vi "Configure Trigger Link.vi"(0 "VISA resource name":refnum<visa-resource-name>, 1 "Trigger Layer Input Port (3)":u32=3, 2 "Trigger Layer Output Port (4)":u32=4, 5 "Arm Layer Input Port (1)":u32=1, 7 "Arm Layer Output Port (2)":u32=2, 9 "Arm Layer Output Events (1)":u32=1, 11 "error in (no error)":errorcluster, 12 "Trigger Layer Input Events (1)":u32=1, 13 "Trigger Layer Output Events (1)":u32=1) -> (4 "VISA resource name out":refnum<visa-resource-name>, 15 "error out":errorcluster)   [LabVIEW 2012, in "Keithley 24XX.lvlib"]
doc: "Configure the trigger link ports as well as the events that require or create a trigger event."
uses:
  <instrlib>/Keithley 24XX/Keithley 24XX.lvlib
panel:
  # "Arm Layer Controls"
  # "Trigger Layer Controls"
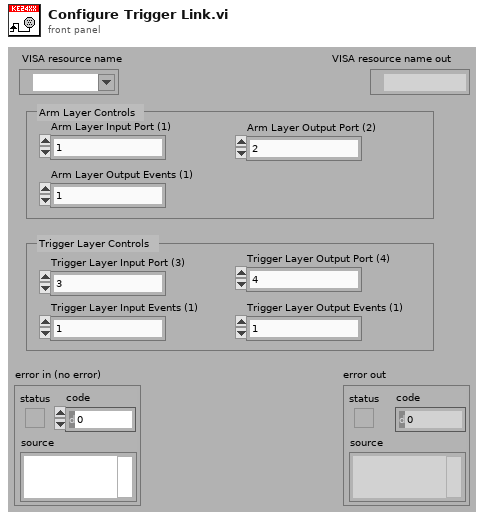
[diagram p1: front panel]
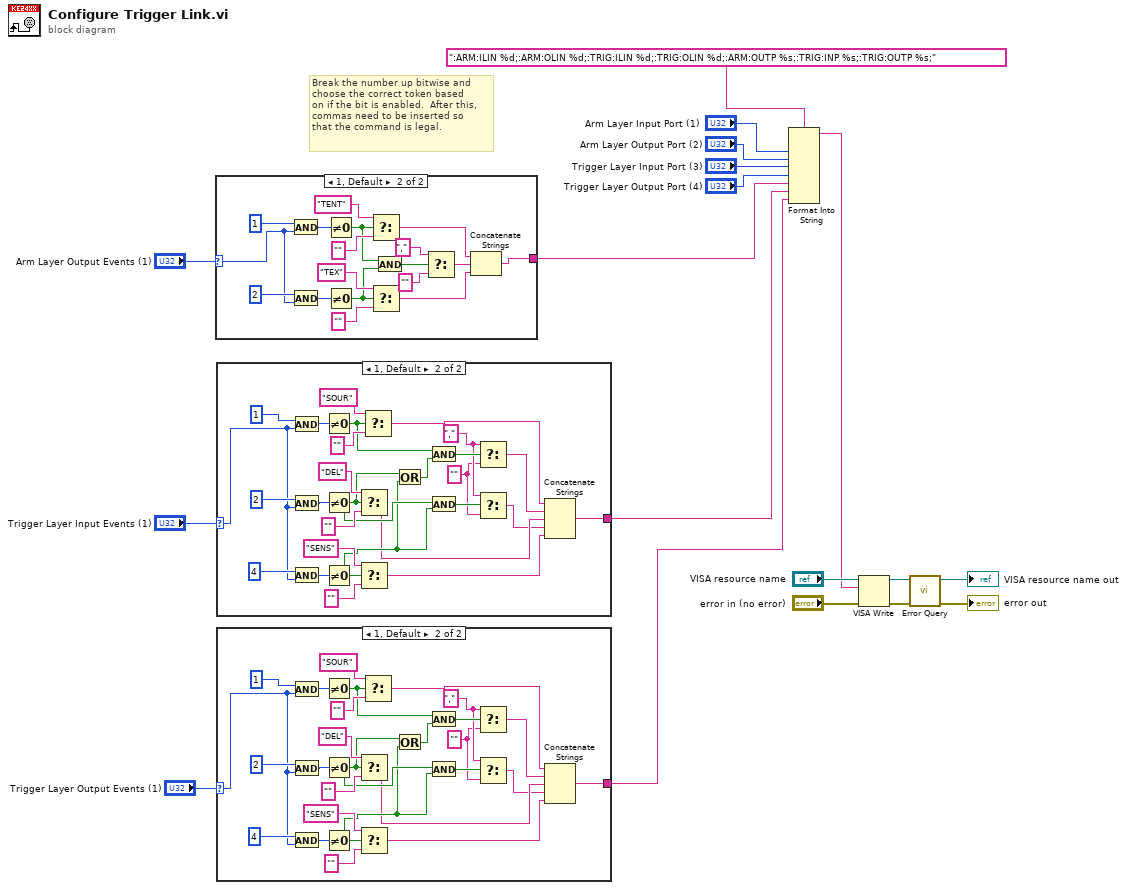
[diagram p0: block diagram]
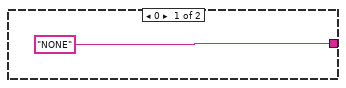
[diagram p2: hidden frame]
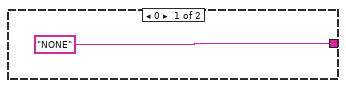
[diagram p3: hidden frame]
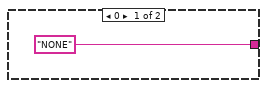
[diagram p4: hidden frame]
diagram:
  # "Break the number up bitwise and\nchoose the correct token based\non if the bit is enabled.  After this, \ncommas need to be inserted so \nthat the command is legal."
  n1 = case shown="1, Default" "Arm Layer Output Events (1)" {
    selector: "Arm Layer Output Events (1)" -> [_ w35]
    tunnel: ["NONE" w20] -> w4
    frame 0 {
    }
    frame 1, Default {
      n2 = And(x=1, y=w35) -> (x .and. y?=w34:u32)
      n3 = And(x=2, y=w35) -> (x .and. y?=w33:u32)
      n4 = Not Equal To 0?(x=w34) -> (x != 0?=w28:bool)
      n5 = Not Equal To 0?(x=w33) -> (x != 0?=w27:bool)
      n6 = Select(t="TENT", s=w28, f="") -> (s? t:f=w21:string)
      n7 = Select(t="TEX", s=w27, f="") -> (s? t:f=w22:string)
      n8 = And(x=w28, y=w27) -> (x .and. y?=w26:bool)
      n9 = Select(t=",", s=w26, f="") -> (s? t:f=w23:string)
      n10 = Concatenate Strings(w21, w23, w22) -> (w20:string)
    }
  }
  n11 = case shown="1, Default" "Trigger Layer Input Events (1)" {
    selector: "Trigger Layer Input Events (1)" -> [_ w62]
    tunnel: ["NONE" w39] -> w3
    frame 0 {
    }
    frame 1, Default {
      w46 = ","
      w45 = ""
      n12 = And(x=1, y=w62) -> (x .and. y?=w60:u32)
      n13 = And(x=2, y=w62) -> (x .and. y?=w61:u32)
      n14 = And(x=4, y=w62) -> (x .and. y?=w59:u32)
      n15 = Not Equal To 0?(x=w60) -> (x != 0?=w52:bool)
      n16 = Not Equal To 0?(x=w61) -> (x != 0?=w50:bool)
      n17 = Not Equal To 0?(x=w59) -> (x != 0?=w49:bool)
      n18 = Select(t="DEL", s=w50, f="") -> (s? t:f=w42:string)
      n19 = Select(t="SENS", s=w49, f="") -> (s? t:f=w40:string)
      n20 = Select(t="SOUR", s=w52, f="") -> (s? t:f=w44:string)
      n21 = Or(x=w50, y=w49) -> (x .or. y?=w51:bool)
      n22 = And(x=w52, y=w51) -> (x .and. y?=w48:bool)
      n23 = And(x=w50, y=w49) -> (x .and. y?=w47:bool)
      n24 = Select(t=w46, s=w48, f=w45) -> (s? t:f=w43:string)
      n25 = Select(t=w46, s=w47, f=w45) -> (s? t:f=w41:string)
      n26 = Concatenate Strings(w44, w43, w42, w41, w40) -> (w39:string)
    }
  }
  n27 = case shown="1, Default" "Trigger Layer Output Events (1)" {
    selector: "Trigger Layer Output Events (1)" -> [_ w90]
    tunnel: ["NONE" w67] -> w1
    frame 0 {
    }
    frame 1, Default {
      w74 = ","
      w73 = ""
      n28 = And(x=1, y=w90) -> (x .and. y?=w88:u32)
      n29 = And(x=2, y=w90) -> (x .and. y?=w89:u32)
      n30 = And(x=4, y=w90) -> (x .and. y?=w87:u32)
      n31 = Not Equal To 0?(x=w88) -> (x != 0?=w80:bool)
      n32 = Not Equal To 0?(x=w89) -> (x != 0?=w78:bool)
      n33 = Not Equal To 0?(x=w87) -> (x != 0?=w77:bool)
      n34 = Select(t="DEL", s=w78, f="") -> (s? t:f=w70:string)
      n35 = Select(t="SENS", s=w77, f="") -> (s? t:f=w68:string)
      n36 = Select(t="SOUR", s=w80, f="") -> (s? t:f=w72:string)
      n37 = Or(x=w78, y=w77) -> (x .or. y?=w79:bool)
      n38 = And(x=w80, y=w79) -> (x .and. y?=w76:bool)
      n39 = And(x=w78, y=w77) -> (x .and. y?=w75:bool)
      n40 = Select(t=w74, s=w76, f=w73) -> (s? t:f=w71:string)
      n41 = Select(t=w74, s=w75, f=w73) -> (s? t:f=w69:string)
      n42 = Concatenate Strings(w72, w71, w70, w69, w68) -> (w67:string)
    }
  }
  n43 = Format Into String(format string=":ARM:ILIN %d;:ARM:OLIN %d;:TRIG:ILIN %d;:TRIG:OLIN %d;:ARM:OUTP %s;:TRIG:INP %s;:TRIG:OUTP %s;", "Arm Layer Input Port (1)", "Arm Layer Output Port (2)", "Trigger Layer Input Port (3)", "Trigger Layer Output Port (4)", w4, w3, w1) -> (resulting string=w6:string)  [unwired: 2 in, 1 out]
  n44 = VISA Write(VISA resource name="VISA resource name", write buffer=w6, error in (no error)="error in (no error)") -> (VISA resource name out=w14:refnum<visa-resource-name>, error out=w13:errorcluster)  [unwired: 1 out]
  n45 = call <instrlib>:"Error Query.vi"("error in (no error)"=w13, "VISA resource name"=w14) -> ("error out"=→"error out":errorcluster, "VISA resource name out"=→"VISA resource name out":refnum<visa-resource-name>)  [unwired: 6 in, 2 out]
